vi "Timer.vi"(8 "error in (no error)":errorcluster, 10 "Timer Command":T1, 11 "Time Target (s)":dbl=1.0) -> (0 "error out":errorcluster, 2 "Time has Elapsed":bool, 3 "Elapsed Time (s)":dbl)   [LabVIEW 2019]
uses:
  Controls/TimerStates.ctl
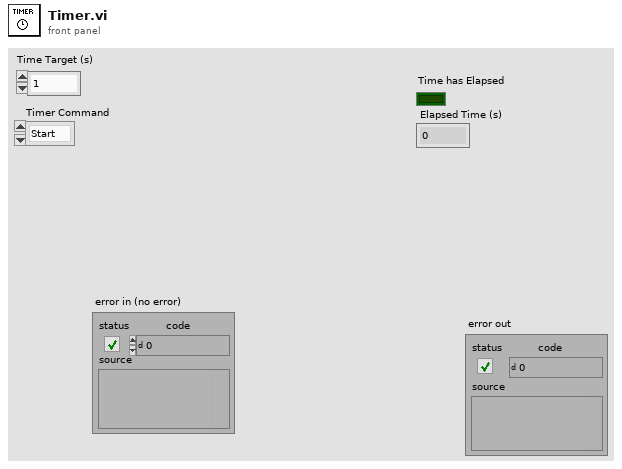
[diagram p1: front panel]
types:
  T1 = typedef "TimerStates.ctl" = enum16{"Start", "Read"}
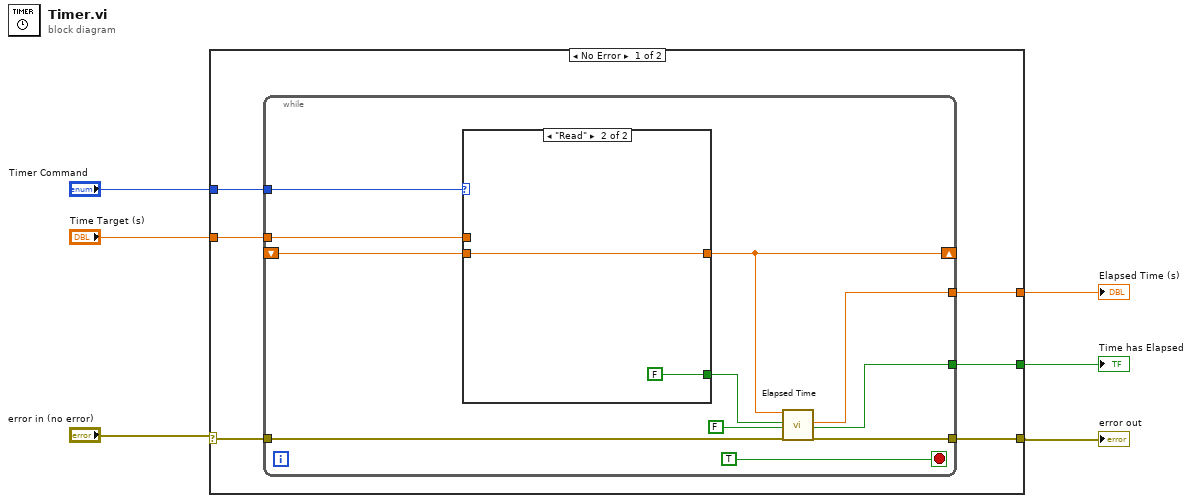
[diagram p0: block diagram]
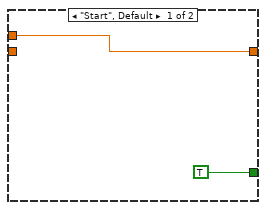
[diagram p2: hidden frame]
diagram:
  n1 = case shown="No Error" "error in (no error)" {
    selector: "error in (no error)" -> [w9 w28]
    tunnel: "Timer Command" -> [w12 _]
    tunnel: [w11 _] -> w5
    tunnel: [w10 _] -> w1
    tunnel: [w8 w28] -> w3
    tunnel: "Time Target (s)" -> [w7 _]
    frame No Error {
      n2 = while {
        tunnel: w12 -> [w22]
        tunnel: w9 -> [w20]
        tunnel: [w18] -> w8
        tunnel: [w19] -> w11
        shift-right: [w15] -> _
        shift-left: _ -> [w17]
        tunnel: w7 -> [w16]
        tunnel: [w14] -> w10
        stop <- TRUE stop-if-true
        n3 = case shown="\"Read\"" w22 {
          tunnel: [TRUE ("Reset") FALSE ("Reset")] -> w21
          tunnel: w17 -> [_ w26]
          tunnel: [w24 w26] -> w15
          tunnel: w16 -> [w24 _]
          frame "Start", Default {
          }
          frame "Read" {
          }
        }
        n4 = call "Elapsed Time"("Time Target (s)"=w15, "Reset"=w21, "Auto Reset"=FALSE, "error in (no error)"=w20) -> ("Elapsed Time (s)"=w14:dbl, "Time has Elapsed"=w19:bool, "error out"=w18:errorcluster)  [unwired: 8 in, 5 out]
      }
    }
    frame Error {
    }
  }
  "Time has Elapsed" <- w5
  "Elapsed Time (s)" <- w1
  "error out" <- w3
